vi "Run Step.vi"(8 "error in (no error)":errorcluster, 9 "result allocation":T1, 10 "parameters":T1, 11 "Numeric Limit Compare in":refnum<class "Numeric Limit Compare.lvclass">) -> (0 "error out":errorcluster, 1 "results":T1, 2 "parameter allocation":T1, 3 "Numeric Limit Compare out":refnum<class "Numeric Limit Compare.lvclass">)   [LabVIEW 2015, in "Numeric Limit Compare.lvclass"]
uses:
  Numeric Limit Compare.lvclass
  <vilib>/NI/Tag Bus/table/data table.ctl
  Numeric Limit Compare.lvclass/Numeric Limit Compare.ctl
  <vilib>/NI/Tag Bus/table/data polymorphs/read one/read Double.vi
  <vilib>/NI/Tag Bus/table/data polymorphs/write one/write Boolean.vi
  <vilib>/NI/Tag Bus/table/data table.lvlib
panel:
  out "Pass/Fail ?":bool
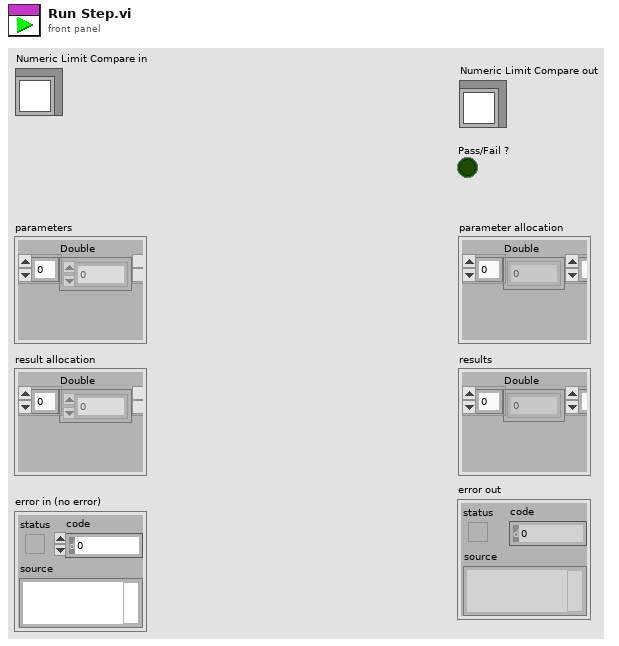
[diagram p1: front panel]
types:
  T1 = typedef "tag bus.lvlib/data table.lvlib/data table.ctl" = cluster{"Double":dbl[], "Single":sgl[], "I64":i64[], "I32":i32[], "I16":i16[], "I8":i8[], "U64":u64[], "U32":u32[], "U16":u16[], "U8":u8[], "Boolean":bool[], "String":string[], "Array of Double":cluster{"DBL Array":dbl[]}[], "Array of Single":cluster{"SGL Array":sgl[]}[], "Array of I64":cluster{"I64 Array":i64[]}[], "Array of I32":cluster{"I32 Array":i32[]}[], "Array of I16":cluster{"I16 Array":i16[]}[], "Array of I8":cluster{"I8 Array":i8[]}[], "Array of U64":cluster{"U64 Array":u64[]}[], "Array of U32":cluster{"U32 Array":u32[]}[], "Array of U16":cluster{"U16 Array":u16[]}[], "Array of U8":cluster{"U8 Array":u8[]}[], "Array of Boolean":cluster{"Boolean Array":bool[]}[], "Array of String":cluster{"String Array":string[]}[]}
  T2 = typedef "Comparison Types.ctl" = enum16{"GELE (>=<=)", "GTLE(><=)", "GTLT(><)", "GELT(>=<)", "EQ(==)", "NE (!=)", "GT(>)", "LT(<)", "GE(>=)", "LE(<=)"}
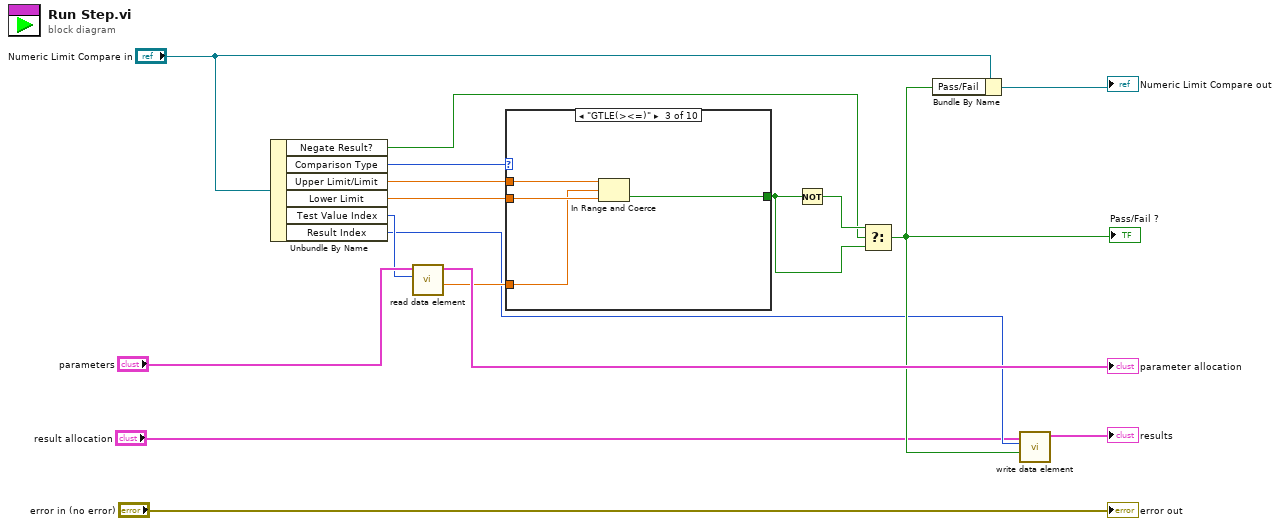
[diagram p0: block diagram]
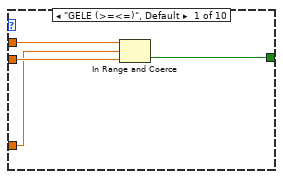
[diagram p2: hidden frame]
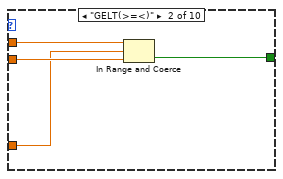
[diagram p3: hidden frame]
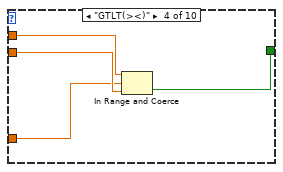
[diagram p4: hidden frame]
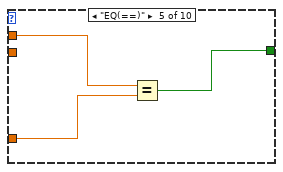
[diagram p5: hidden frame]
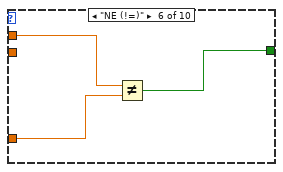
[diagram p6: hidden frame]
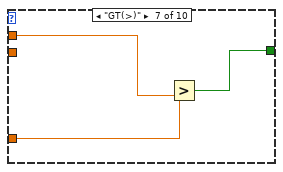
[diagram p7: hidden frame]
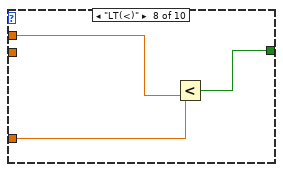
[diagram p8: hidden frame]
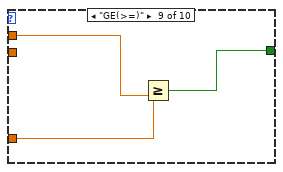
[diagram p9: hidden frame]
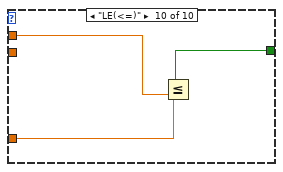
[diagram p10: hidden frame]
diagram:
  n1 = Unbundle By Name("Numeric Limit Compare in") -> ("Negate Result?"=w12:bool, "Comparison Type"=w13:T2, "Upper Limit/Limit"=w11:dbl, "Lower Limit"=w10:dbl, "Test Value Index"=w7:i32, "Result Index"=w3:i32)
  n2 = call-poly <vilib>:"read data element.vi"("index"=w7, "data table in"="parameters") -> ("value"=w9:dbl, "data table out"=→"parameter allocation":T1)  [unwired: 8 in]
  n3 = case shown="\"GTLE(><=)\"" w13 {
    tunnel: w11 -> [w21 w25 w29 w32 w35 w38 w42 w44 w47 w50]
    tunnel: w10 -> [w20 w24 w28 w31 _ _ _ _ _ _]
    tunnel: [w19 w23 w27 w33 w34 w37 w40 w43 w46 w49] -> w15
    tunnel: w9 -> [w18 w22 w26 w30 w36 w39 w41 w45 w48 w51]
    frame "GELE (>=<=)", Default {
      n4 = In Range and Coerce(upper limit=w21, x=w18, lower limit=w20) -> (In Range?=w19:bool)  [unwired: 1 out]
    }
    frame "GELT(>=<)" {
      n5 = In Range and Coerce(upper limit=w25, x=w22, lower limit=w24) -> (In Range?=w23:bool)  [unwired: 1 out]
    }
    frame "GTLE(><=)" {
      n6 = In Range and Coerce(upper limit=w29, x=w26, lower limit=w28) -> (In Range?=w27:bool)  [unwired: 1 out]
    }
    frame "GTLT(><)" {
      n7 = In Range and Coerce(upper limit=w32, x=w30, lower limit=w31) -> (In Range?=w33:bool)  [unwired: 1 out]
    }
    frame "EQ(==)" {
      n8 = Equal?(x=w35, y=w36) -> (x = y?=w34:bool)
    }
    frame "NE (!=)" {
      n9 = Not Equal?(x=w38, y=w39) -> (x != y?=w37:bool)
    }
    frame "GT(>)" {
      n10 = Greater?(x=w41, y=w42) -> (0:w40:bool)
    }
    frame "LT(<)" {
      n11 = Less?(x=w45, y=w44) -> (x < y?=w43:bool)
    }
    frame "GE(>=)" {
      n12 = Greater Or Equal?(x=w48, y=w47) -> (x >= y?=w46:bool)
    }
    frame "LE(<=)" {
      n13 = Less Or Equal?(x=w51, y=w50) -> (x <= y?=w49:bool)
    }
  }
  n14 = Not(x=w15) -> (.not. x?=w14:bool)
  n15 = Select(t=w14, s=w12, f=w15) -> (s? t:f=w4:bool)
  "Pass/Fail ?" <- w4
  n16 = Bundle By Name(cluster="Numeric Limit Compare in", "Pass/Fail"=w4) -> (→"Numeric Limit Compare out":refnum<class "Numeric Limit Compare.lvclass">)
  n17 = call-poly <vilib>:"write data element.vi"("value"=w4, "index"=w3, "data table in"="result allocation") -> ("data table out"=→"results":T1)  [unwired: 8 in]
  "error out" <- "error in (no error)"
